vi "Report Oximetry Set-Rev1.vi"(9 "Spectral Data In":T5={"PDT Amp [v]"=0.0, "RIS Amp [v]"=0.0, "B-Field"=[], "All In-Phase Scan Spectra"=[], "Model Select"=enum."OneCompRISTwoPDT", "Fit Each Scan"=FALSE, "PDT Center [g]"=0.0, "In-Phase Average Spectra"=[], "In-Phase Median Spectra"=[], "Out-Phase Median Spectra"=[], "Out-Phase Average Spectra"=[], "Fit Spectra"=[], "Fit No-Baseline Spectra"=[], "All Out-Phase Scan Spectra"=[], "Baseline Offset Correction"=FALSE, "In-Phase Offset [v]"=0.0, "Out-Phase Offset [v]"=0.0, "Ch2 Input\n(Balance)"=[], "Ch3 Input\n(Phase)"=[], "Ch4 Input\n(AFC)"=[], "Fit Pars"=[], "Fit Pars Errors"=[], "Fit Pars Labels"=[], "Raw Scan DAQ Data"=[], "Bad Scans Indicies"=[], "Good In-Phase Scan Spectra"=[], "Good Out-Phase Scan Spectra"=[], "Bad In-Phase Scan Spectra"=[], "Bad Out-Phase Scan Spectra"=[], "Number of bad scans"=0, "Fit History"=[], "PDT Amp. History/Set [v]"=[], "RIS Amp. History/Set [v]"=[], "RIS Amp. History/Scan [v]"=[], "All Shifted B-Fields"=[], "Good Shifted B-Fields"=[], "Ch5 Input\n(SpO2)"=[], "Ch6 Input\n(BPM)"=[], "Global SNR"=0.0, "Fit Error History"=[], "SNR History"=[]} {"Global SNR" min=0.0; "PDT Center [g]" min=0.0; "RIS Amp [v]" min=0.0}, 10 "Measurement Information In":T2={"Comments"="", "Directory Input"="", "Data file path"=path "C:/Data/EPR Data", "Scripting File"=path "C:/Data/Configuration Script.csv", "Save Data"=FALSE, "Tooth size (d11) [mm]"=0.0, "Tooth size (d12) [mm]"=0.0, "Tooth size (d21) [mm]"=0.0, "Tooth size (d22) [mm]"=0.0, "Dose of Tooth [Gy]"=0.0, "Safe Shutdown?"=FALSE, "Gases Available"=[], "Database Username"="", "Database Password"="", "Database Login URL"="", "Database Upload URL"="", "Database Success URL"="", "Database XML URL"="", "Database Resonator URL"="", "Session Number"=0, "Set #"=0, "Resonator Operator"="", "Session Type"="", "Tooth/Sample ID"="", "Volunteer ID"="", "Computer Operator"="", "Volunteer Type"="", "Site/Tooth Selection (T8,T9)"="", "Resonator"="", "Measurement Site"="", "Non-standard session?"=FALSE, "EPR DAQ Version"="", "Session Path"=path "C:/Data/EPR Data", "Chosen Applied State"="", "Chosen Initial State"="", "Time of Transition"="", "DAQ Mode"=enum."Engineering", "pO2/Scan [mmHg]"=[], "pO2/Set [mmHg]"=[], "Linewidth (HWHM)/Scan [Gauss]"=[], "Linewidth (HWHM)/Set [Gauss]"=[], "pO2 Conversion"="", "Dose Calibration Cluster"={"Dose Response"={"grand_mean"=0.0292016, "slope"=0.0188720543}, "Dose Correction"={"Sex"=1, "a0"=7.719669421, "a1"=-2.746550736, "a2"=-0.186490355, "a3"=0.041922063, "a4"=-0.849147359, "a5"=0.14330063, "a6"=0.019930219, "A_n"=40.0, "H_n"=10.12, "Dose Correction"=FALSE}, "Dose Reporting"={"Reporting is"=TRUE, "sd_threshold [AU]"=0.06, "sd_model [Gy]"=0.66, "dosimetric_threshold [Gy]"=2.0, "Add intrasession errors is"=FALSE, "Prior Radiation?"=FALSE}}, "OxyChip Slope"=0.0, "OxyChip Intercept"=0.0, "QA Mode"=enum."Select QA Mode", "QA Session?"=FALSE, "Sample Type"=enum."Empty Resonator", "Report pO2/Scan"=FALSE, "Skip End Session Save"=FALSE, "Number of sites"=enum."# Probes", "Recipient Name"="", "Sender Name"="", "Recipient Email"="", "Transition State History"=[], "pO2 Report Times"=[], "Temperature [C]"=0.0, "+Error pO2/Scan [mmHg]"=[], "-Error pO2/Scan [mmHg]"=[], "+Error pO2/Set [mmHg]"=[], "-Error pO2/Set [mmHg]"=[], "Oxy Phase Exclusion Tolerance [rad]"=0.0, "Oxy Center Exclusion Tolerance [%]"=0.0, "Oxy Exclude Unacceptable"=FALSE, "Oxy Unacceptable Estimate Flags"=[], "Save Session PPT"=FALSE, "Flagged Bad Sets"=[]} {"Oxy Center Exclusion Tolerance [%]" format="%#_9g"; "Oxy Phase Exclusion Tolerance [rad]" format="%#_9g"; "Temperature [C]" format="%#_9g"; "OxyChip Intercept" format="%#_9g"; "OxyChip Slope" format="%#_9g"; "Dose Calibration Cluster"."Dose Reporting"."dosimetric_threshold [Gy]" format="%#_9g"; "Dose Calibration Cluster"."Dose Reporting"."sd_model [Gy]" format="%#_9g"; "Dose Calibration Cluster"."Dose Reporting"."sd_threshold [AU]" format="%#_9g"; "Dose Calibration Cluster"."Dose Correction"."H_n" format="%#_9g"; "Dose Calibration Cluster"."Dose Correction"."A_n" format="%#_9g"; "Dose Calibration Cluster"."Dose Correction"."a6" format="%#.9g"; "Dose Calibration Cluster"."Dose Correction"."a5" format="%#.9g"; "Dose Calibration Cluster"."Dose Correction"."a4" format="%#.9g"; "Dose Calibration Cluster"."Dose Correction"."a3" format="%#.9g"; "Dose Calibration Cluster"."Dose Correction"."a2" format="%#.9g"; "Dose Calibration Cluster"."Dose Correction"."a1" format="%#.9g"; "Dose Calibration Cluster"."Dose Correction"."a0" format="%#.9g"; "Dose Calibration Cluster"."Dose Correction"."Sex" items=["Male"=1, "Female"=0]; "Dose Calibration Cluster"."Dose Response"."slope" format="%#_9g"; "Dose Calibration Cluster"."Dose Response"."grand_mean" format="%#_9g"}, 11 "Acquisition Parameters In":T1={"Magnet Angle [deg]"=0.0, "Magnet Angles [deg]"=[], "DeltaVpp [v]"=0.0, "SEM [v]"=0.0, "DeltaVpp Thresh [v]"=0.0, "SEM Thresh [v]"=0.0, "Adaptive Processing"=FALSE, "Acquire Q"=FALSE, "Acquire Photos"=FALSE, "Adaptive Tuning"=FALSE, "Automated Matching"=FALSE, "X-Gradient [G/mm]"=0.0, "Y-Gradient [G/mm]"=0.0, "Z-Gradient [G/mm]"=0.0, "Central Field [G]"=0.0, "Scan Width [G]"=0.0, "Mod. Amp. [G]"=0.0, "Scan Time [s]"=0.0, "Pre-Scan Delay [ms]"=0, "Measurement Timeout [s]"=0.0, "Electromagnet Main Field [G]"=0.0, "Locked Central Field [G]"=0.0, "Scans Excluded"=0, "Scans Completed"=0, "No. Scans/Set"=0, "No. Scans for SNR"=0, "Field Locked Frequency [GHz]"=0.0, "Auto Set-based Field Center"=FALSE, "Prompt for oxy acquisition updates"=FALSE, "Oxy QA Scan?"=FALSE, "Exclude Bad Data"=FALSE, "Optimizing RF Power"=FALSE, "Gradients on/off"=TRUE, "Running Script"=FALSE, "Opto-Coupler Current [A]"=0.0, "Continuous Sweeping"=FALSE, "Sweep Rise Time [sec]"=0, "Reverse Sweep Central Field [G]"=0.0, "Forward Sweep Central Field [G]"=0.0, "Sweep Calibrated"=FALSE, "Modulation Calibrated"=FALSE, "First CheckCal Scan?"=FALSE, "AFC Field Correction"=FALSE, "OxyQAInit Scan Width [G]"=0.0, "OxyQAInit Mod. Amp. [G]"=0.0, "Scans Completed/Session"=0, "Acquire SpO2"=FALSE, "Acquire Temperature"=FALSE, "Over Mod"=FALSE} {"OxyQAInit Mod. Amp. [G]" min=0.0; "OxyQAInit Scan Width [G]" min=0.0; "Mod. Amp. [G]" min=0.0; "Scan Width [G]" min=0.0; "Measurement Timeout [s]" min=0.0; "Scan Time [s]" min=0.0; "Z-Gradient [G/mm]" min=0.0; "Y-Gradient [G/mm]" min=0.0; "X-Gradient [G/mm]" min=0.0; "SEM Thresh [v]" min=0.0; "DeltaVpp Thresh [v]" min=0.0; "SEM [v]" min=0.0}) -> (0 "Report pO2":bool, 2 "Measurement Information Out":T2={"Comments"="", "Directory Input"="", "Data file path"=path "C:/Data/EPR Data", "Scripting File"=path "C:/Data/Configuration Script.csv", "Save Data"=FALSE, "Tooth size (d11) [mm]"=0.0, "Tooth size (d12) [mm]"=0.0, "Tooth size (d21) [mm]"=0.0, "Tooth size (d22) [mm]"=0.0, "Dose of Tooth [Gy]"=0.0, "Safe Shutdown?"=FALSE, "Gases Available"=[], "Database Username"="", "Database Password"="", "Database Login URL"="", "Database Upload URL"="", "Database Success URL"="", "Database XML URL"="", "Database Resonator URL"="", "Session Number"=0, "Set #"=0, "Resonator Operator"="", "Session Type"="", "Tooth/Sample ID"="", "Volunteer ID"="", "Computer Operator"="", "Volunteer Type"="", "Site/Tooth Selection (T8,T9)"="", "Resonator"="", "Measurement Site"="", "Non-standard session?"=FALSE, "EPR DAQ Version"="", "Session Path"=path "C:/Data/EPR Data", "Chosen Applied State"="", "Chosen Initial State"="", "Time of Transition"="", "DAQ Mode"=enum."Engineering", "pO2/Scan [mmHg]"=[], "pO2/Set [mmHg]"=[], "Linewidth (HWHM)/Scan [Gauss]"=[], "Linewidth (HWHM)/Set [Gauss]"=[], "pO2 Conversion"="", "Dose Calibration Cluster"={"Dose Response"={"grand_mean"=0.0292016, "slope"=0.0188720543}, "Dose Correction"={"Sex"=1, "a0"=7.719669421, "a1"=-2.746550736, "a2"=-0.186490355, "a3"=0.041922063, "a4"=-0.849147359, "a5"=0.14330063, "a6"=0.019930219, "A_n"=40.0, "H_n"=10.12, "Dose Correction"=FALSE}, "Dose Reporting"={"Reporting is"=TRUE, "sd_threshold [AU]"=0.06, "sd_model [Gy]"=0.66, "dosimetric_threshold [Gy]"=2.0, "Add intrasession errors is"=FALSE, "Prior Radiation?"=FALSE}}, "OxyChip Slope"=0.0, "OxyChip Intercept"=0.0, "QA Mode"=enum."Select QA Mode", "QA Session?"=FALSE, "Sample Type"=enum."Empty Resonator", "Report pO2/Scan"=FALSE, "Skip End Session Save"=FALSE, "Number of sites"=enum."# Probes", "Recipient Name"="", "Sender Name"="", "Recipient Email"="", "Transition State History"=[], "pO2 Report Times"=[], "Temperature [C]"=0.0, "+Error pO2/Scan [mmHg]"=[], "-Error pO2/Scan [mmHg]"=[], "+Error pO2/Set [mmHg]"=[], "-Error pO2/Set [mmHg]"=[], "Oxy Phase Exclusion Tolerance [rad]"=0.0, "Oxy Center Exclusion Tolerance [%]"=0.0, "Oxy Exclude Unacceptable"=FALSE, "Oxy Unacceptable Estimate Flags"=[], "Save Session PPT"=FALSE, "Flagged Bad Sets"=[]} {"Oxy Center Exclusion Tolerance [%]" format="%#_9g"; "Oxy Phase Exclusion Tolerance [rad]" format="%#_9g"; "Temperature [C]" format="%#_9g"; "OxyChip Intercept" format="%#_9g"; "OxyChip Slope" format="%#_9g"; "Dose Calibration Cluster"."Dose Reporting"."dosimetric_threshold [Gy]" format="%#_9g"; "Dose Calibration Cluster"."Dose Reporting"."sd_model [Gy]" format="%#_9g"; "Dose Calibration Cluster"."Dose Reporting"."sd_threshold [AU]" format="%#_9g"; "Dose Calibration Cluster"."Dose Correction"."H_n" format="%#_9g"; "Dose Calibration Cluster"."Dose Correction"."A_n" format="%#_9g"; "Dose Calibration Cluster"."Dose Correction"."a6" format="%#.9g"; "Dose Calibration Cluster"."Dose Correction"."a5" format="%#.9g"; "Dose Calibration Cluster"."Dose Correction"."a4" format="%#.9g"; "Dose Calibration Cluster"."Dose Correction"."a3" format="%#.9g"; "Dose Calibration Cluster"."Dose Correction"."a2" format="%#.9g"; "Dose Calibration Cluster"."Dose Correction"."a1" format="%#.9g"; "Dose Calibration Cluster"."Dose Correction"."a0" format="%#.9g"; "Dose Calibration Cluster"."Dose Correction"."Sex" items=["Male"=1, "Female"=0]; "Dose Calibration Cluster"."Dose Response"."slope" format="%#_9g"; "Dose Calibration Cluster"."Dose Response"."grand_mean" format="%#_9g"})   [LabVIEW 2016]
uses:
  Types/Measurement Information.ctl
  Dose Calculation and Reporting/Dose Calculation Control.ctl
  Types/Sample Type.ctl
  Types/Spectral Data.ctl
  Types/Fitting Model Selection.ctl
  Types/Acquisition Parameters.ctl
panel:
  # "Gradients"
  # "Field"
  # "Scans and Sets"
  # "Timing"
  # "Adaptive Dosimetric \nData Processing"
  # "Session Information"
  # "Oximetric Data and Information"
  # "Email"
  # "Tooth Information"
  # "Database"
  # "Session Information"
  # "Oximetric Data and Information"
  # "Email"
  # "Tooth Information"
  # "Database"
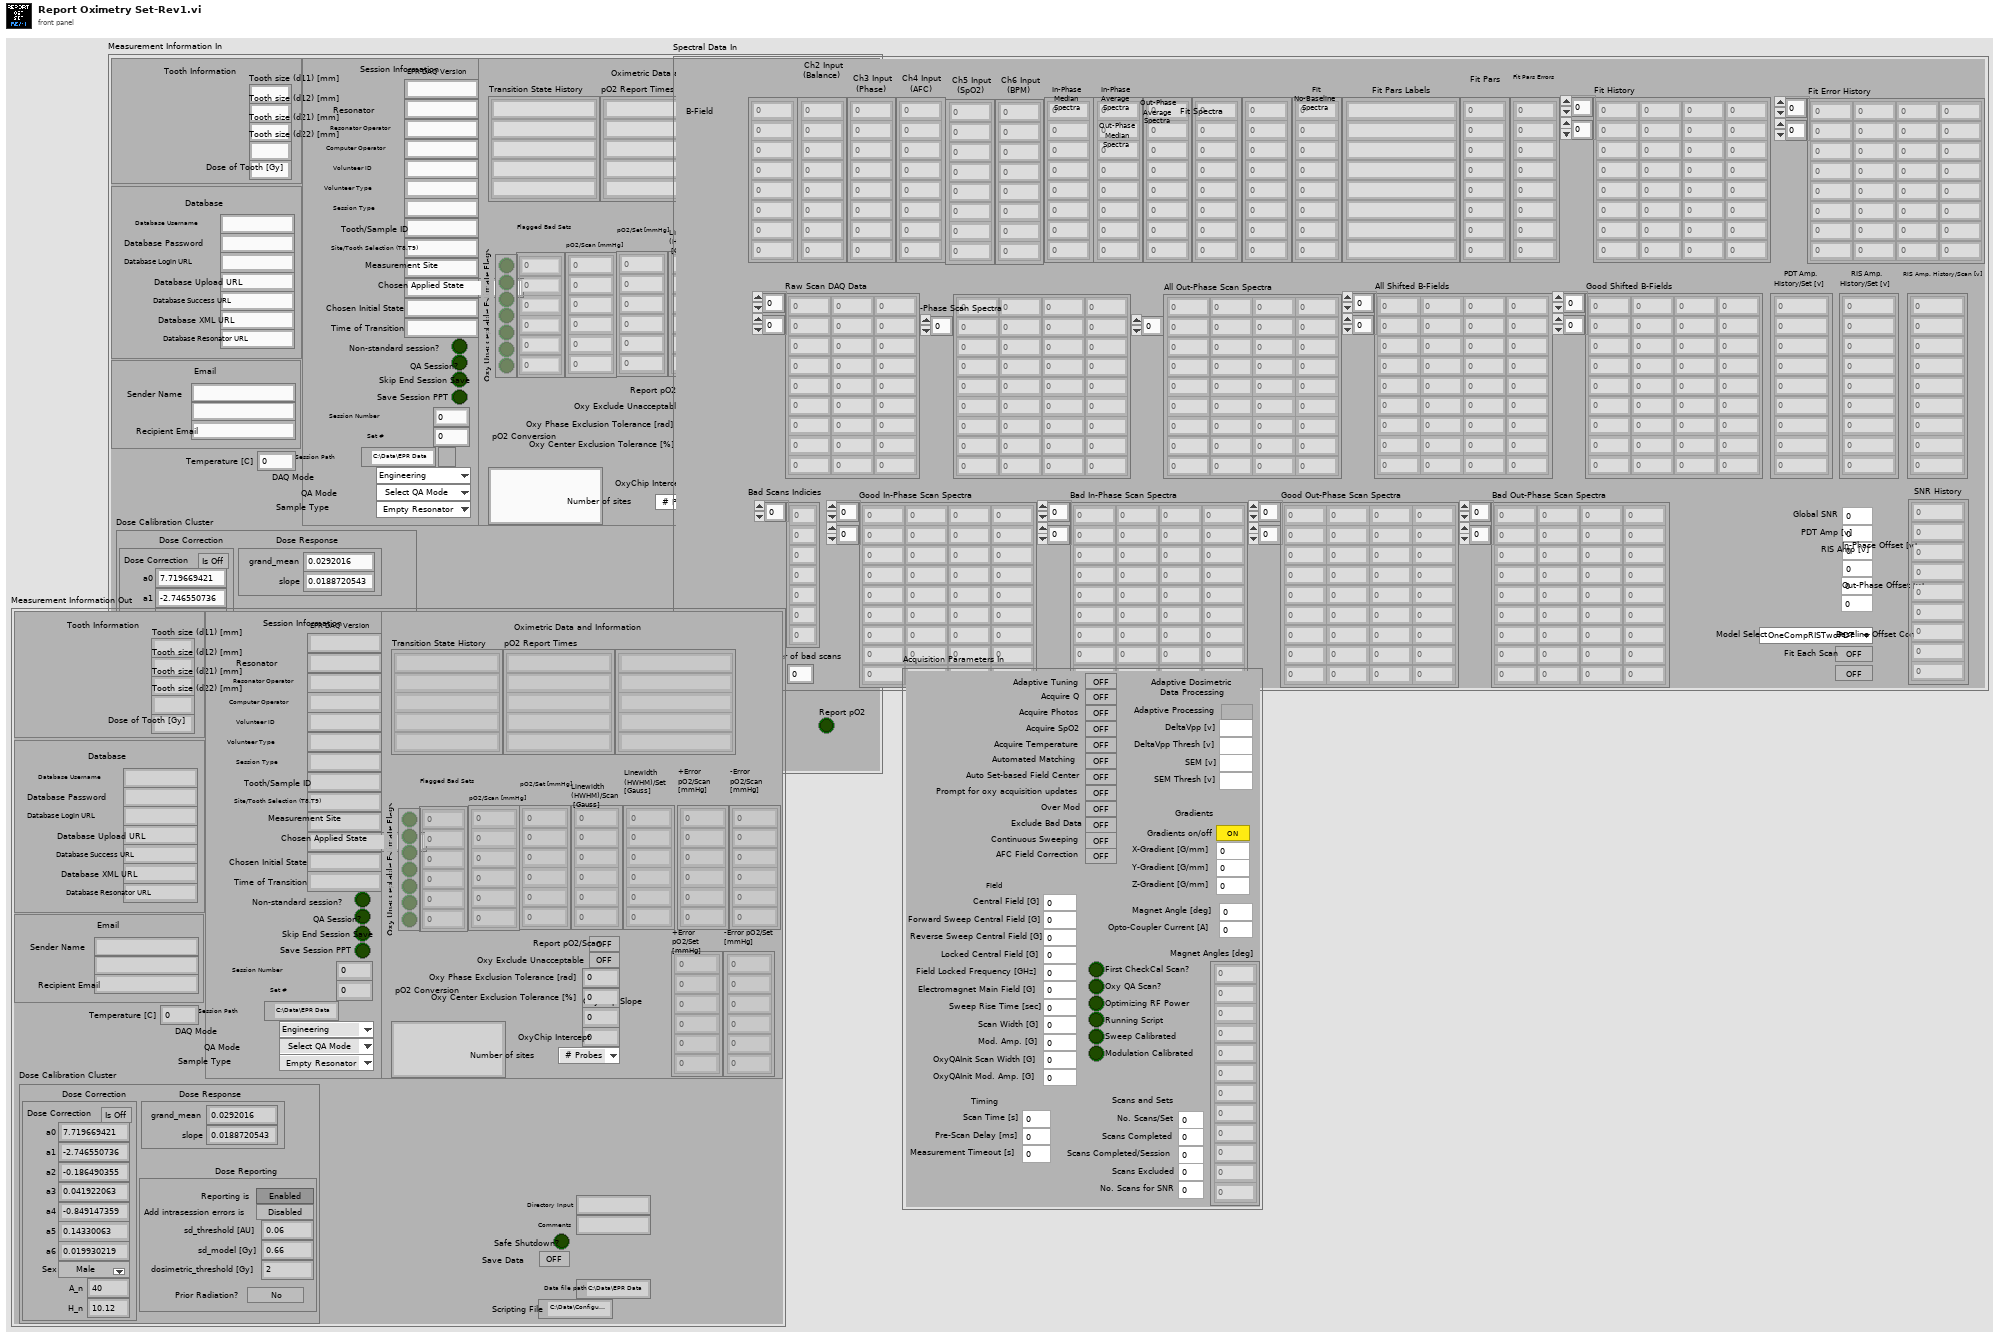
[diagram p1: front panel]
types:
  T1 = typedef "Acquisition Parameters.ctl" = cluster{"Magnet Angle [deg]":dbl, "Magnet Angles [deg]":dbl[], "DeltaVpp [v]":dbl, "SEM [v]":dbl, "DeltaVpp Thresh [v]":dbl, "SEM Thresh [v]":dbl, "Adaptive Processing":bool, "Acquire Q":bool, "Acquire Photos":bool, "Adaptive Tuning":bool, "Automated Matching":bool, "X-Gradient [G/mm]":dbl, "Y-Gradient [G/mm]":dbl, "Z-Gradient [G/mm]":dbl, "Central Field [G]":dbl, "Scan Width [G]":dbl, "Mod. Amp. [G]":dbl, "Scan Time [s]":dbl, "Pre-Scan Delay [ms]":u32, "Measurement Timeout [s]":dbl, "Electromagnet Main Field [G]":dbl, "Locked Central Field [G]":dbl, "Scans Excluded":u32, "Scans Completed":u32, "No. Scans/Set":u32, "No. Scans for SNR":u32, "Field Locked Frequency [GHz]":dbl, "Auto Set-based Field Center":bool, "Prompt for oxy acquisition updates":bool, "Oxy QA Scan?":bool, "Exclude Bad Data":bool, "Optimizing RF Power":bool, "Gradients on/off":bool, "Running Script":bool, "Opto-Coupler Current [A]":dbl, "Continuous Sweeping":bool, "Sweep Rise Time [sec]":u32, "Reverse Sweep Central Field [G]":dbl, "Forward Sweep Central Field [G]":dbl, "Sweep Calibrated":bool, "Modulation Calibrated":bool, "First CheckCal Scan?":bool, "AFC Field Correction":bool, "OxyQAInit Scan Width [G]":dbl, "OxyQAInit Mod. Amp. [G]":dbl, "Scans Completed/Session":u32, "Acquire SpO2":bool, "Acquire Temperature":bool, "Over Mod":bool}
  T2 = typedef "Measurement Information.ctl" = cluster{"Comments":string, "Directory Input":string, "Data file path":path, "Scripting File":path, "Save Data":bool, "Tooth size (d11) [mm]":dbl, "Tooth size (d12) [mm]":dbl, "Tooth size (d21) [mm]":dbl, "Tooth size (d22) [mm]":dbl, "Dose of Tooth [Gy]":dbl, "Safe Shutdown?":bool, "Gases Available":string[], "Database Username":string, "Database Password":string, "Database Login URL":string, "Database Upload URL":string, "Database Success URL":string, "Database XML URL":string, "Database Resonator URL":string, "Session Number":i32, "Set #":u32, "Resonator Operator":string, "Session Type":string, "Tooth/Sample ID":string, "Volunteer ID":string, "Computer Operator":string, "Volunteer Type":string, "Site/Tooth Selection (T8,T9)":string, "Resonator":string, "Measurement Site":string, "Non-standard session?":bool, "EPR DAQ Version":string, "Session Path":path, "Chosen Applied State":string, "Chosen Initial State":string, "Time of Transition":string, "DAQ Mode":enum16{"Engineering", "Dosimetry", "Oximetry"}, "pO2/Scan [mmHg]":dbl[][], "pO2/Set [mmHg]":dbl[][], "Linewidth (HWHM)/Scan [Gauss]":dbl[][], "Linewidth (HWHM)/Set [Gauss]":dbl[][], "pO2 Conversion":string, "Dose Calibration Cluster":T3, "OxyChip Slope":dbl, "OxyChip Intercept":dbl, "QA Mode":enum16{"Select QA Mode", "QA-Start/End", "QA-Mid", "QA-Weekly", "QA-Eng", "Check Calibration"}, "QA Session?":bool, "Sample Type":T4, "Report pO2/Scan":bool, "Skip End Session Save":bool, "Number of sites":enum16{"# Probes", "1", "2", "3", "4"}, "Recipient Name":string, "Sender Name":string, "Recipient Email":string, "Transition State History":string[], "pO2 Report Times":string[], "Temperature [C]":dbl, "+Error pO2/Scan [mmHg]":dbl[][], "-Error pO2/Scan [mmHg]":dbl[][], "+Error pO2/Set [mmHg]":dbl[][], "-Error pO2/Set [mmHg]":dbl[][], "Oxy Phase Exclusion Tolerance [rad]":dbl, "Oxy Center Exclusion Tolerance [%]":dbl, "Oxy Exclude Unacceptable":bool, "Oxy Unacceptable Estimate Flags":bool[], "Save Session PPT":bool, "Flagged Bad Sets":u32[]}
  T3 = typedef "Dose Calculation Control.ctl" = cluster{"Dose Response":cluster{"grand_mean":dbl, "slope":dbl}, "Dose Correction":cluster{"Sex":u16, "a0":dbl, "a1":dbl, "a2":dbl, "a3":dbl, "a4":dbl, "a5":dbl, "a6":dbl, "A_n":dbl, "H_n":dbl, "Dose Correction":bool}, "Dose Reporting":cluster{"Reporting is":bool, "sd_threshold [AU]":dbl, "sd_model [Gy]":dbl, "dosimetric_threshold [Gy]":dbl, "Add intrasession errors is":bool, "Prior Radiation?":bool}}
  T4 = typedef "Sample Type.ctl" = enum16{"Empty Resonator", "IRS", "BallZero", "Irradiated Tooth", "Non-irradiated Tooth", "OxyChip", "LiPc", "PDT", "India Ink"}
  T5 = typedef "Spectral Data.ctl" = cluster{"PDT Amp [v]":dbl, "RIS Amp [v]":dbl, "B-Field":dbl[], "All In-Phase Scan Spectra":dbl[][], "Model Select":T6, "Fit Each Scan":bool, "PDT Center [g]":dbl, "In-Phase Average Spectra":dbl[], "In-Phase Median Spectra":dbl[], "Out-Phase Median Spectra":dbl[], "Out-Phase Average Spectra":dbl[], "Fit Spectra":dbl[], "Fit No-Baseline Spectra":dbl[], "All Out-Phase Scan Spectra":dbl[][], "Baseline Offset Correction":bool, "In-Phase Offset [v]":dbl, "Out-Phase Offset [v]":dbl, "Ch2 Input\n(Balance)":dbl[], "Ch3 Input\n(Phase)":dbl[], "Ch4 Input\n(AFC)":dbl[], "Fit Pars":dbl[], "Fit Pars Errors":dbl[], "Fit Pars Labels":string[], "Raw Scan DAQ Data":dbl[][], "Bad Scans Indicies":i32[], "Good In-Phase Scan Spectra":dbl[][], "Good Out-Phase Scan Spectra":dbl[][], "Bad In-Phase Scan Spectra":dbl[][], "Bad Out-Phase Scan Spectra":dbl[][], "Number of bad scans":i32, "Fit History":dbl[][], "PDT Amp. History/Set [v]":dbl[], "RIS Amp. History/Set [v]":dbl[], "RIS Amp. History/Scan [v]":dbl[], "All Shifted B-Fields":dbl[][], "Good Shifted B-Fields":dbl[][], "Ch5 Input\n(SpO2)":dbl[], "Ch6 Input\n(BPM)":dbl[], "Global SNR":dbl, "Fit Error History":dbl[][], "SNR History":dbl[]}
  T6 = typedef "Fitting Model Selection.ctl" = enum16{"OneCompRIS", "OneCompRISTwoPDT", "OneCompRISRev", "OneCompRISTwoPDTRev", "LiPc", "TwoLiPc", "ThreeLiPc", "FourLiPc", "PDTCalibration", "CE_Ink", "Printex", "MelaninTwoPDT"}
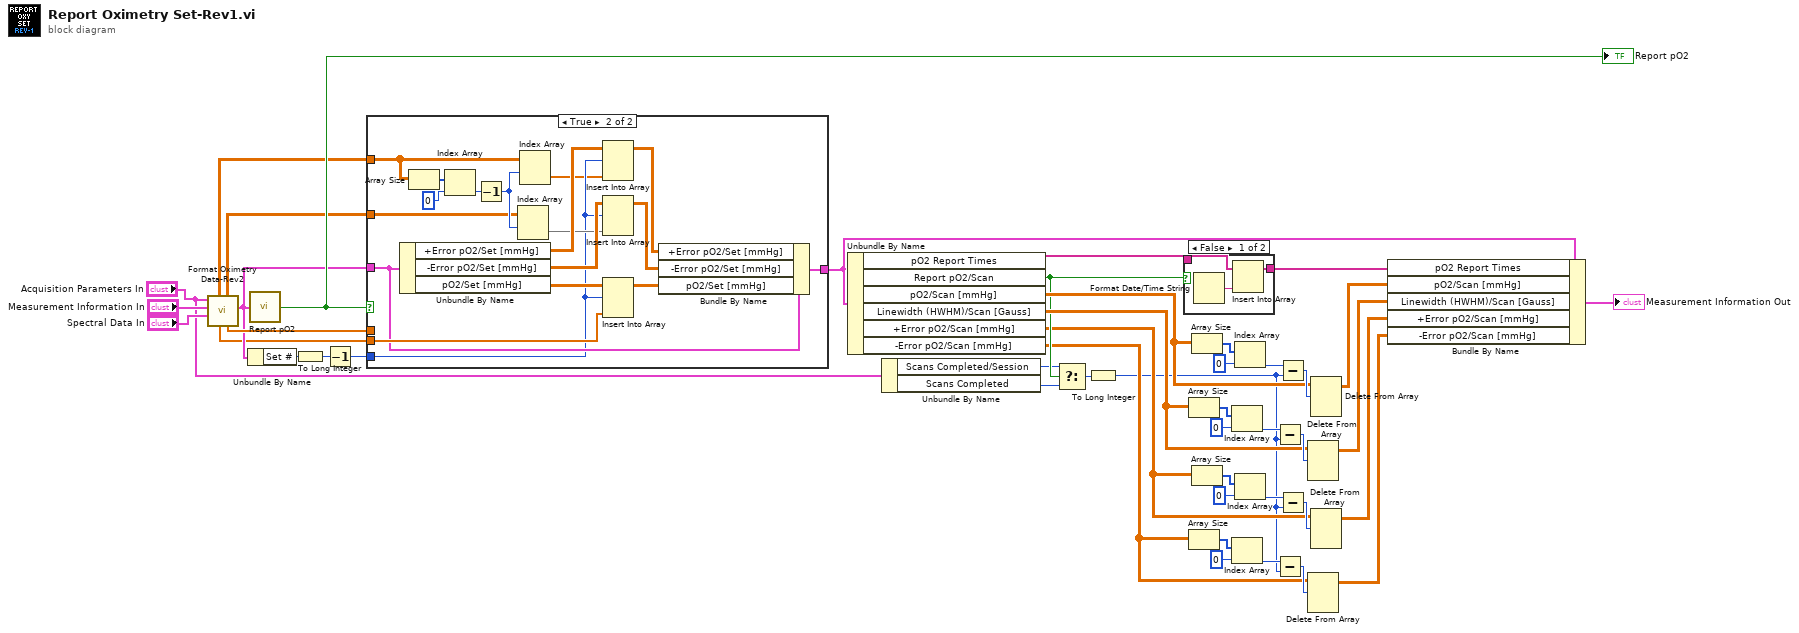
[diagram p0: block diagram]
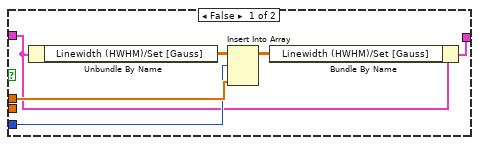
[diagram p3: hidden frame]
diagram:
  n1 = call "Format Oximetry Data-Rev2.vi"("Spectral Data In"="Spectral Data In", "Measurement Information In"="Measurement Information In", "Acquisition Parameters In"="Acquisition Parameters In") -> ("Measurement Information Out"=w41:T2, "Calibration dBpp [Gauss]"=w43:dbl[], "Negative pO2 Error [mmHg]"=w1:dbl[][], "pO2 [mmHg]"=w40:dbl[], "Positive pO2 Error [mmHg]"=w2:dbl[][])  [unwired: 2 in, 2 out]
  n2 = Unbundle By Name(w41) -> ("Set #"=w38:u32)
  n3 = call "Report pO2.vi"("Measurement Information"=w41) -> ("Report pO2"=w44:bool)
  "Report pO2" <- w44
  n4 = To Long Integer(number=w38) -> (32bit integer=w39:i32)
  n5 = Decrement(x=w39) -> (x-1=w37:i32)
  n6 = case shown="True" w44 {
    tunnel: w43 -> [w51 _]
    tunnel: w37 -> [w50 w55]
    tunnel: w41 -> [w48 w66]
    tunnel: [w46 w65] -> w33
    tunnel: w40 -> [_ w67]
    tunnel: w2 -> [_ w60]
    tunnel: w1 -> [_ w59]
    frame False {
      n7 = Unbundle By Name(w48) -> ("Linewidth (HWHM)/Set [Gauss]"=w49:dbl[][])
      n8 = Insert Into Array(array=w49, index (row)=w50, new element=w51) -> (w47:dbl[][])  [unwired: 1 in]
      n9 = Bundle By Name(cluster=w48, "Linewidth (HWHM)/Set [Gauss]"=w47) -> (w46:T2)
    }
    frame True {
      n10 = Unbundle By Name(w66) -> ("+Error pO2/Set [mmHg]"=w58:dbl[][], "-Error pO2/Set [mmHg]"=w57:dbl[][], "pO2/Set [mmHg]"=w69:dbl[][])
      n11 = Array Size(array=w60) -> (size(s)=w64:i32[])
      n12 = Index Array(array=w64, index=0) -> (element=w62:i32)
      n13 = Decrement(x=w62) -> (x-1=w61:i32)
      n14 = Index Array(array=w59, index (row)=w61) -> (element=w56:dbl[])  [unwired: 1 in]
      n15 = Index Array(array=w60, index (row)=w61) -> (element=w52:dbl[])  [unwired: 1 in]
      n16 = Insert Into Array(array=w58, index (row)=w55, new element=w52) -> (w54:dbl[][])  [unwired: 1 in]
      n17 = Insert Into Array(array=w57, index (row)=w55, new element=w56) -> (w53:dbl[][])  [unwired: 1 in]
      n18 = Insert Into Array(array=w69, index (row)=w55, new element=w67) -> (w68:dbl[][])  [unwired: 1 in]
      n19 = Bundle By Name(cluster=w66, "+Error pO2/Set [mmHg]"=w54, "-Error pO2/Set [mmHg]"=w53, "pO2/Set [mmHg]"=w68) -> (w65:T2)
    }
  }
  n20 = Unbundle By Name(w33) -> ("pO2 Report Times"=w36:string[], "Report pO2/Scan"=w19:bool, "pO2/Scan [mmHg]"=w24:dbl[][], "Linewidth (HWHM)/Scan [Gauss]"=w23:dbl[][], "+Error pO2/Scan [mmHg]"=w7:dbl[][], "-Error pO2/Scan [mmHg]"=w6:dbl[][])
  n21 = Unbundle By Name("Acquisition Parameters In") -> ("Scans Completed/Session"=w17:u32, "Scans Completed"=w16:u32)
  n22 = Select(t=w17, s=w19, f=w16) -> (s? t:f=w18:u32)
  n23 = To Long Integer(number=w18) -> (32bit integer=w5:i32)
  n24 = case shown="False" w19 {
    tunnel: w36 -> [w72 w73]
    tunnel: [w70 w73] -> w35
    frame False {
      n25 = Format Date/Time String() -> (date/time string=w71:string)  [unwired: 3 in]
      n26 = Insert Into Array(array=w72, new element=w71) -> (w70:string[])  [unwired: 1 in]
    }
    frame True {
    }
  }
  n27 = Array Size(array=w23) -> (size(s)=w26:i32[])
  n28 = Array Size(array=w6) -> (size(s)=w14:i32[])
  n29 = Array Size(array=w24) -> (size(s)=w30:i32[])
  n30 = Array Size(array=w7) -> (size(s)=w10:i32[])
  n31 = Index Array(array=w26, index=0) -> (element=w28:i32)
  n32 = Index Array(array=w14, index=0) -> (element=w12:i32)
  n33 = Index Array(array=w30, index=0) -> (element=w32:i32)
  n34 = Index Array(array=w10, index=0) -> (element=w8:i32)
  n35 = Subtract(x=w28, y=w5) -> (x-y=w25:i32)
  n36 = Subtract(x=w12, y=w5) -> (x-y=w15:i32)
  n37 = Subtract(x=w32, y=w5) -> (x-y=w29:i32)
  n38 = Subtract(x=w8, y=w5) -> (x-y=w11:i32)
  n39 = Delete From Array(array=w23, length=w25) -> (array with subset deleted=w20:dbl[][])  [unwired: 2 in, 1 out]
  n40 = Delete From Array(array=w6, length=w15) -> (array with subset deleted=w3:dbl[][])  [unwired: 2 in, 1 out]
  n41 = Delete From Array(array=w24, length=w29) -> (array with subset deleted=w21:dbl[][])  [unwired: 2 in, 1 out]
  n42 = Delete From Array(array=w7, length=w11) -> (array with subset deleted=w4:dbl[][])  [unwired: 2 in, 1 out]
  n43 = Bundle By Name(cluster=w33, "pO2 Report Times"=w35, "pO2/Scan [mmHg]"=w21, "Linewidth (HWHM)/Scan [Gauss]"=w20, "+Error pO2/Scan [mmHg]"=w4, "-Error pO2/Scan [mmHg]"=w3) -> (→"Measurement Information Out":T2)
